vi "v1.9 trying to make it modular.vi"() -> ()   [LabVIEW 2018]
uses:
  <vilib>/Analysis/baseanly.llb/Mean (DBL).vi
  <vilib>/DAQmx/read.llb/DAQmx Read (Analog 1D DBL NChan 1Samp).vi
  <extravilib>/ChannelInstances/High Speed Stream-a[.](dbl)/_Read For Replicate.vi
  <vilib>/DAQmx/create/channels.llb/DAQmx Create Channel (AI-Voltage-Basic).vi
  <vilib>/DAQmx/configure/timing.llb/DAQmx Timing (Sample Clock).vi
  <extravilib>/ChannelInstances/High Speed Stream-a[.](dbl)/Instantiate.vi
  <extravilib>/ChannelInstances/High Speed Stream-a[.](dbl)/)Channel.vi
  <extravilib>/ChannelInstances/High Speed Stream-a[.](dbl)/Abort Signal/Init Signal.vi
  <vilib>/DAQmx/miscellaneous.llb/DAQmx Fill In Error Info.vi
  <extravilib>/ChannelInstances/High Speed Stream-a[.](dbl).lvlib
  <vilib>/Analysis/NI_AALBase.lvlib
panel:
  in  "stop 3":bool
  in  "stop 2":bool
  in  "stop":bool
  in  "Avg Of?":dbl
  in  "Record?":bool
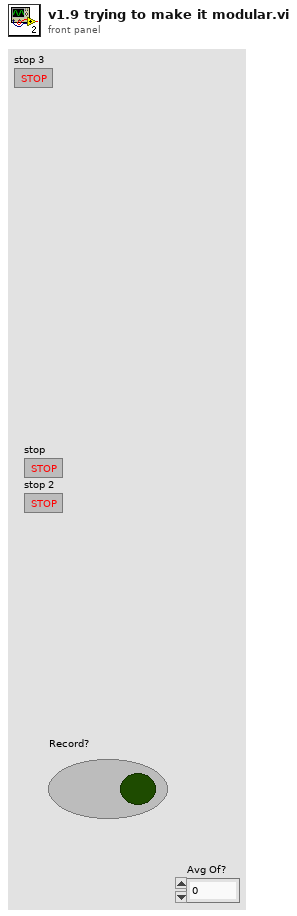
[diagram p1: front panel]
types:
  T1 = typedef "High Speed Stream-a[.](dbl).lvlib/)Channel.ctl" = refnum<queue>
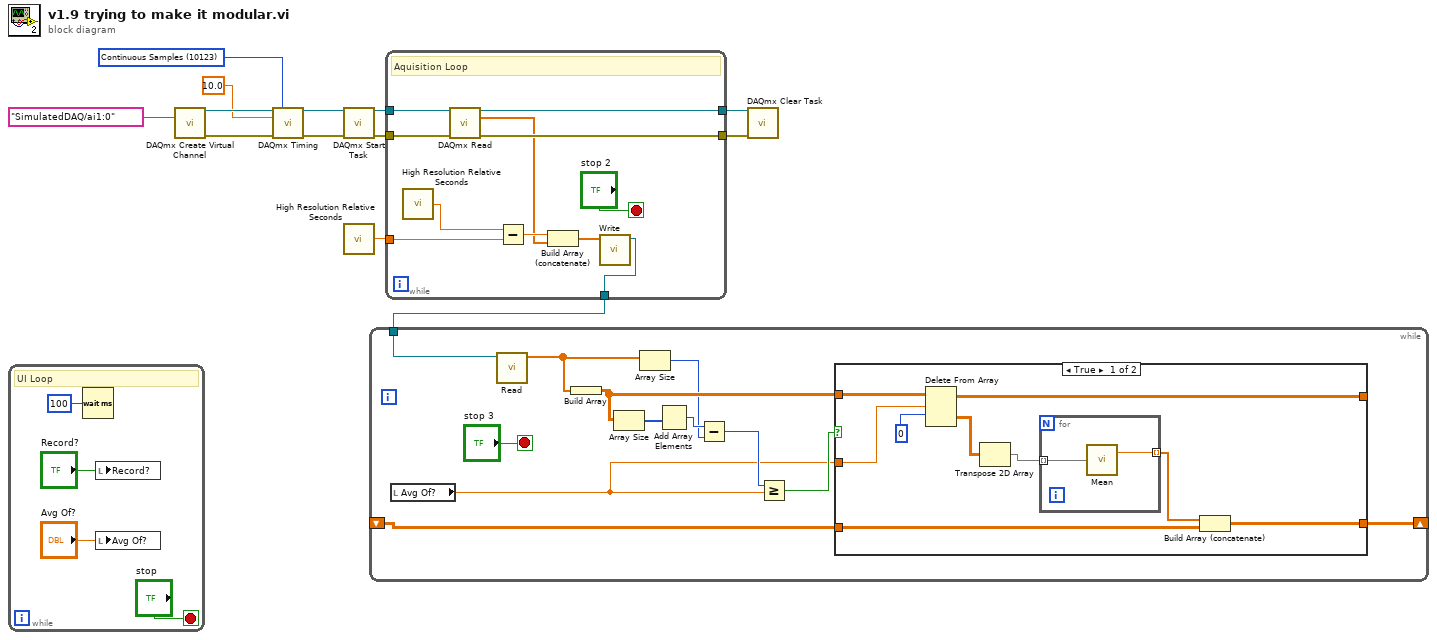
[diagram p0: block diagram]
diagram:
  w9 = 10123 items=["Finite Samples"=10178, "Continuous Samples"=10123, "Hardware Timed Single Point"=12522] ("sample mode")
  n1 = while {
    stop <- "stop" stop-if-true
    # "UI Loop"
    n2 = Wait (ms)(milliseconds to wait=u32 100) -> ()  [unwired: 1 out]
    n3 = local write "Record?"("Record?") -> ()
    n4 = local write "Avg Of?"("Avg Of?") -> ()
  }
  n5 = call-poly <vilib>:"DAQmx Create Virtual Channel.vi"("physical channels"=tag "SimulatedDAQ/ai1:0") -> ("task out"=w10:refnum<k21>, "error out"=w11:errorcluster)  [unwired: 13 in]
  n6 = call-poly <vilib>:"DAQmx Timing.vi"("task/channels in"=w10, "sample mode"=w9, "rate"=10.0, "error in"=w11) -> ("task out"=w12:refnum<k21>, "error out"=w13:errorcluster)  [unwired: 10 in]
  n7 = call <vilib>:"DAQmx Start Task.vi"("task/channels in"=w12, "error in"=w13) -> ("task out"=w3:refnum<k21>, "error out"=w4:errorcluster)  [unwired: 12 in]
  n8 = call <vilib>:"High Resolution Relative Seconds.vi"() -> ("relative seconds"=w2:dbl)
  n9 = while {
    tunnel: w3 -> [w25]
    tunnel: w4 -> [w28]
    tunnel: [w27] -> w7
    tunnel: [w26] -> w6
    tunnel: w2 -> [w22]
    tunnel: [w18] -> w1
    stop <- "stop 2" stop-if-true
    # "Aquisition Loop"
    n10 = call <vilib>:"High Resolution Relative Seconds.vi"() -> ("relative seconds"=w23:dbl)
    n11 = call-poly <vilib>:"DAQmx Read.vi"("task/channels in"=w25, "error in"=w28) -> ("task out"=w27:refnum<k21>, "data"=w20:dbl[], "error out"=w26:errorcluster)  [unwired: 11 in]
    n12 = Subtract(x=w23, y=w22) -> (x-y=w21:dbl)
    n13 = Build Array (concatenate)(w21, w20) -> (w19:dbl[])
    n14 = call <extravilib>:"Write.vi"("element"=w19) -> ("channel"=w18:T1)  [unwired: 8 in, 2 out]
  }
  n15 = while {
    shift-right: [w33] -> _
    shift-left: _ -> [w32]
    tunnel: w1 -> [w31]
    stop <- "stop 3" stop-if-true
    n16 = local read "Avg Of?"() -> (w34:dbl)
    n17 = call <extravilib>:"Read.vi"("channel"=w31) -> ("element"=w30:dbl[])  [unwired: 6 in, 4 out]
    n18 = Build Array(w30) -> (w40:dbl[][])
    n19 = Array Size(array=w40) -> (size(s)=w39:i32[])
    n20 = Array Size(array=w30) -> (size(s)=w37:i32)
    n21 = Add Array Elements(numeric array=w39) -> (sum=w38:i32)
    n22 = Subtract(x=w38, y=w37) -> (x-y=w35:i32)
    n23 = Greater Or Equal?(x=w35, y=w34) -> (x >= y?=w36:bool)
    n24 = case shown="True" w36 {
      tunnel: [w46 w53] -> _
      tunnel: w40 -> [w49 w53]
      tunnel: w34 -> [w48 _]
      tunnel: [w42 w52] -> w33
      tunnel: w32 -> [w41 w52]
      frame True {
        n25 = Delete From Array(array=w49, length=w48, index (row)=0) -> (deleted portion=w45:dbl[][], array with subset deleted=w46:dbl[][])  [unwired: 1 in]
        n26 = Transpose 2D Array(2D array=w45) -> (transposed array=w44:dbl[][])
        n27 = for {
          tunnel: w44 -> [w51] mode=indexing
          tunnel: [w50] -> w43 mode=indexing
          n28 = call-poly <vilib>:"Mean.vi"("X"=w51) -> ("mean"=w50:dbl)  [unwired: 1 out]
        }
        n29 = Build Array (concatenate)(w43, w41) -> (w42:dbl[][])
      }
      frame False {
      }
    }
  }
  n30 = call <vilib>:"DAQmx Clear Task.vi"("task in"=w7, "error in"=w6) -> ()  [unwired: 13 in, 1 out]
